vi "Yaw control.vi"(7 "Control Cluster":T1, 8 "error in (no error)":errorcluster, 10 "Target yaw (deg)":sgl, 11 "NavData In":T2) -> (0 "error out":errorcluster, 3 "Control Cluster Out":T1)   [LabVIEW 2014]
uses:
  <vilib>/LVH/AR Drone Toolkit/Decode NavData/Typedefs/NavData Demo.ctl
  <vilib>/LVH/AR Drone Toolkit/AR Drone.lvlib
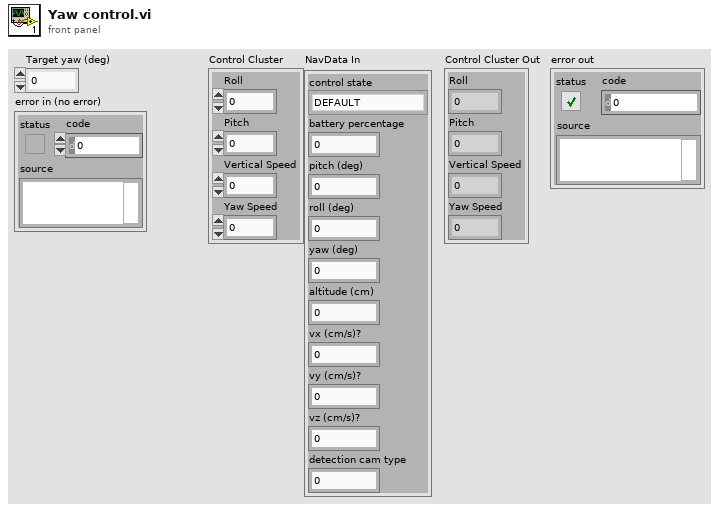
[diagram p1: front panel]
types:
  T1 = cluster{"Roll":sgl, "Pitch":sgl, "Vertical Speed":sgl, "Yaw Speed":sgl}
  T2 = typedef "AR Drone.lvlib/NavData Demo.ctl" = cluster{"control state":enum32{"DEFAULT", "INIT", "LANDING", "FLYING", "HOVERING", "TEST", "TRANS_TAKEOFF", "TRANS_GOTOFIX", "TRANS_LANDING"}, "battery percentage":u32, "pitch (deg)":sgl, "roll (deg)":sgl, "yaw (deg)":sgl, "altitude (cm)":u32, "vx (cm/s)?":sgl, "vy (cm/s)?":sgl, "vz (cm/s)?":sgl, "detection cam type":u32}
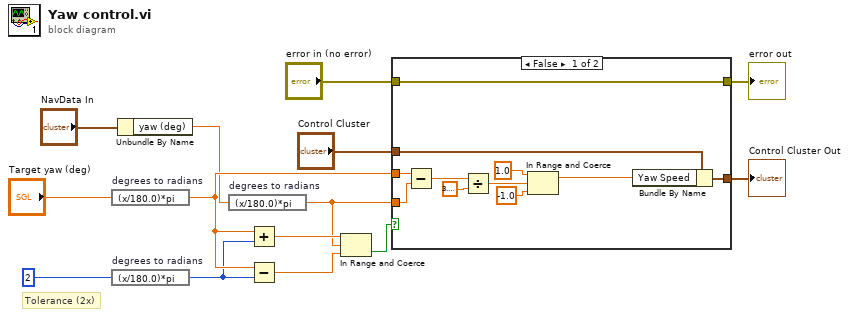
[diagram p0: block diagram]
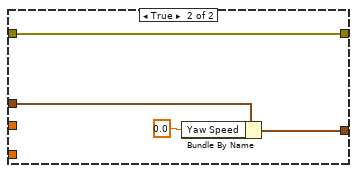
[diagram p2: hidden frame]
diagram:
  # "Tolerance (2x)"
  n1 = expression code="(x/180.0)*pi" "degrees to radians"("Target yaw (deg)") -> (w5:sgl)
  n2 = expression code="(x/180.0)*pi" "degrees to radians"(2) -> (w2:i32)
  n3 = Unbundle By Name("NavData In") -> ("yaw (deg)"=w4:sgl)
  n4 = expression code="(x/180.0)*pi" "degrees to radians"(w4) -> (w1:sgl)
  n5 = Add(x=w5, y=w2) -> (x+y=w12:sgl)
  n6 = Subtract(x=w5, y=w2) -> (x-y=w13:sgl)
  n7 = In Range and Coerce(upper limit=w12, x=w1, lower limit=w13) -> (In Range?=w11:bool)  [unwired: 1 out]
  n8 = case shown="False" w11 {
    tunnel: [w25 w28] -> w10
    tunnel: "Control Cluster" -> [w24 w29]
    tunnel: "error in (no error)" -> [w16 w26]
    tunnel: [w16 w26] -> w7
    tunnel: w1 -> [w22 _]
    tunnel: w5 -> [w23 _]
    frame False {
      n9 = Subtract(x=w23, y=w22) -> (x-y=w18:sgl)
      n10 = Divide(x=w18, y=3.141592653589793) -> (x/y=w17:dbl)
      n11 = In Range and Coerce(upper limit=1.0, x=w17, lower limit=-1.0) -> (coerced(x)=w21:dbl)  [unwired: 1 out]
      n12 = Bundle By Name(cluster=w24, "Yaw Speed"=w21) -> (w25:T1)
    }
    frame True {
      n13 = Bundle By Name(cluster=w29, "Yaw Speed"=sgl 0.0) -> (w28:T1)
    }
  }
  "Control Cluster Out" <- w10
  "error out" <- w7
